vi "PCO_LensControl.vi"() -> (1 "Raw_Length":u16, 4 "Length":u16, 6 "PCO_LensControl_Raw_x64":T2, 7 "PCO_LensControl_Raw_win32":T3, 8 "PCO_LensControl":T1)   [LabVIEW 2019, in "SDK.lvlib" / "Structures.lvlib"]
doc: "Use this template to build a VI to use as a subVI."
uses:
  Structures.lvlib
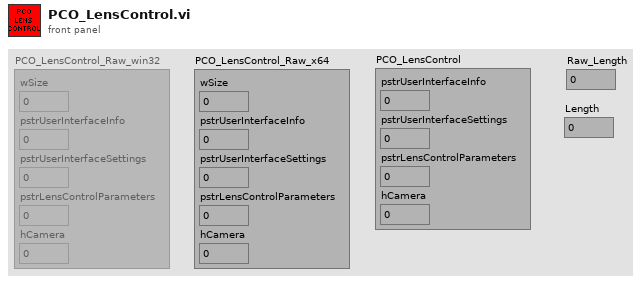
[diagram p1: front panel]
types:
  T1 = cluster{"pstrUserInterfaceInfo":u64, "pstrUserInterfaceSettings":u64, "pstrLensControlParameters":u64, "hCamera":u64}
  T2 = cluster{"wSize":u16, "pstrUserInterfaceInfo":u64, "pstrUserInterfaceSettings":u64, "pstrLensControlParameters":u64, "hCamera":u64}
  T3 = cluster{"wSize":u16, "pstrUserInterfaceInfo":u32, "pstrUserInterfaceSettings":u32, "pstrLensControlParameters":u32, "hCamera":u32}
  T4 = enum8{"Enabled", "Disabled", "Disabled and Grayed Out"}
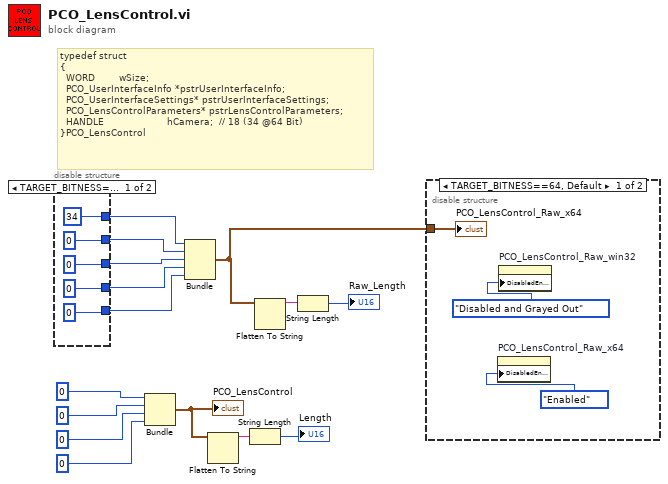
[diagram p0: block diagram]
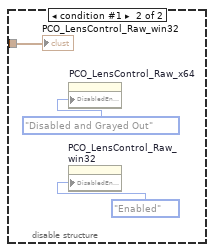
[diagram p2: hidden frame]
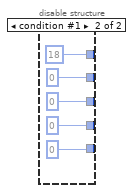
[diagram p3: hidden frame]
diagram:
  # "typedef struct\n{\n  WORD        wSize;\n  PCO_UserInterfaceInfo *pstrUserInterfaceInfo;\n  PCO_UserInterfaceSettings* pstrUserInterfaceSettings;\n  PCO_LensControlParameters* pstrLensControlParameters;\n  HANDLE                     hCamera;  // 18 (34 @64 Bit)\n}PCO_LensControl"
  n1 = disable-structure "Diagram Disable Structure" shown="TARGET_BITNESS==64, Standard" {
    disable-tunnel: [u16 34 ("wSize") u16 18 ("wSize")] -> w10
    disable-tunnel: [u64 0 ("pstrUserInterfaceInfo") u32 0 ("pstrUserInterfaceInfo")] -> w9
    disable-tunnel: [u64 0 ("pstrUserInterfaceSettings") u32 0 ("pstrUserInterfaceSettings")] -> w8
    disable-tunnel: [u64 0 ("pstrLensControlParameters") u32 0 ("pstrLensControlParameters")] -> w7
    disable-tunnel: [u64 0 ("hCamera") u32 0 ("hCamera")] -> w6
    frame condition #0 (active) {
    }
    frame condition #1 {
    }
  }
  n2 = Bundle("pstrUserInterfaceInfo"=u64 0, "pstrUserInterfaceSettings"=u64 0, "pstrLensControlParameters"=u64 0, "hCamera"=u64 0) -> (w11:T1)  [unwired: 1 in]
  "PCO_LensControl" <- w11
  n3 = Bundle("wSize"=w10, "pstrUserInterfaceInfo"=w9, "pstrUserInterfaceSettings"=w8, "pstrLensControlParameters"=w7, "hCamera"=w6) -> (w5:T2)  [unwired: 1 in]
  n4 = Flatten To String(anything=w11) -> (data string=w15:string)  [unwired: 3 in, 2 out]
  n5 = String Length(string=w15) -> (length=→"Length":i32)
  n6 = Flatten To String(anything=w5) -> (data string=w14:string)  [unwired: 3 in, 2 out]
  n7 = String Length(string=w14) -> (length=→"Raw_Length":i32)
  n8 = disable-structure "Diagram Disable Structure" shown="TARGET_BITNESS==64, Default" {
    disable-tunnel: w5 -> [w27 w30]
    frame condition #0 (active) {
      n9 = property on="PCO_LensControl_Raw_x64" class="Clust (strict)"("DisabledEnum"=T4."Enabled" ("Deaktiviert")) -> ()  [unwired: 2 in, 2 out]
      n10 = property on="PCO_LensControl_Raw_win32" class="Clust (strict)"("DisabledEnum"=T4."Disabled and Grayed Out" ("Deaktiviert")) -> ()  [unwired: 2 in, 2 out]
      "PCO_LensControl_Raw_x64" <- w27
    }
    frame condition #1 {
      n11 = property on="PCO_LensControl_Raw_x64" class="Clust (strict)"("DisabledEnum"=T4."Disabled and Grayed Out" ("Deaktiviert")) -> ()  [unwired: 2 in, 2 out]
      n12 = property on="PCO_LensControl_Raw_win32" class="Clust (strict)"("DisabledEnum"=T4."Enabled" ("Deaktiviert")) -> ()  [unwired: 2 in, 2 out]
      "PCO_LensControl_Raw_win32" <- w30
    }
  }
